vi "easing_QuintIn.vi"(9 "distance":dbl, 10 "interval (10 ms)":dbl, 11 "time":dbl) -> (3 "current position":dbl)   [LabVIEW 2023]
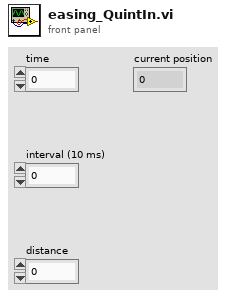
[diagram p1: front panel]
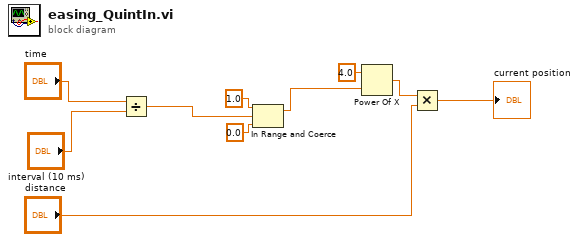
[diagram p0: block diagram]
diagram:
  n1 = Divide(x="time", y="interval (10 ms)") -> (x/y=w2:dbl)
  n2 = In Range and Coerce(upper limit=1.0, x=w2, lower limit=0.0 ("upper limit")) -> (coerced(x)=w1:dbl)  [unwired: 1 out]
  n3 = Power Of X(1:w1, 2:4.0 ("y")) -> (0:w8:dbl)
  n4 = Multiply(x=w8, y="distance") -> (x*y=→"current position":dbl)
